vi "Load Settings from XML.vi"() -> (0 "error out":errorcluster, 3 "Settings out":T1)   [LabVIEW 2025, in "Settings Editor.lvlib"]
doc: "Attempts to load previous user specified settings from an XML file.\n\nThis VI will not generate an error. If a suitable XML file can't be loaded and parsed then it will simply return the default settings.\n_____\nBased on DQMH Dev Tools: Project Template 7.1.0.1503."
uses:
  Settings Editor.lvlib
  Settings--cluster.ctl
  <vilib>/Utility/xml.llb/Read From XML File(string).vi
  Test Meta Data.ctl
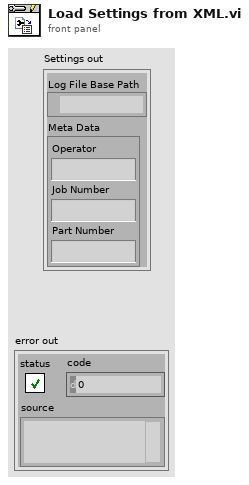
[diagram p1: front panel]
types:
  T1 = typedef "Settings Editor.lvlib/Settings--cluster.ctl" = cluster{"Log File Base Path":path, "Meta Data":T2}
  T2 = typedef "Test Meta Data.ctl" = cluster{"Operator":string, "Job Number":string, "Part Number":string}
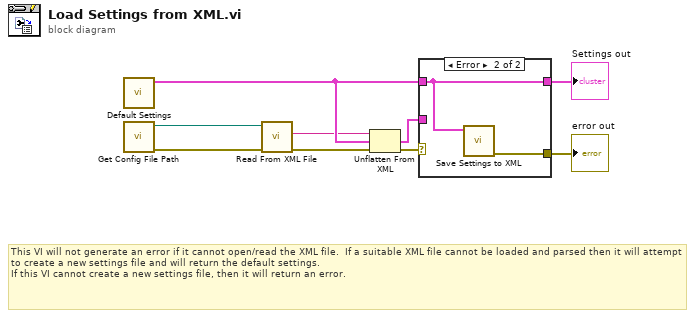
[diagram p0: block diagram]
diagram:
  # "This VI will not generate an error if it cannot open/read the XML file.  If a suitable XML file cannot be loaded and parsed then it will attempt to create a new settings file and will return the default settings.\nIf this VI cannot create a new settings file, then it will return an error."
  n1 = call "Default Settings.vi"() -> ("Default Settings"=w7:T1)  [unwired: 11 in]
  n2 = call "Get Config File Path.vi"() -> ("error out"=w3:errorcluster, "XML File Path"=w4:path)  [unwired: 10 in]
  n3 = call-poly <vilib>:"Read From XML File.vi"("error in (no error)"=w3, "XML File Path"=w4) -> ("error out"=w5:errorcluster, "XML Elements"=w6:string)  [unwired: 7 in, 1 out]
  n4 = Unflatten From XML(xml string=w6, type=w7, error in (no error)=w5) -> (value=w1:T1, error out=w2:errorcluster)
  n5 = case shown="Error" w2 {
    tunnel: [w10 w12] -> w8
    tunnel: w7 -> [_ w12]
    tunnel: w1 -> [w10 _]
    tunnel: [_ w11] -> w9
    frame No Error {
    }
    frame Error {
      n6 = call "Save Settings to XML.vi"("Settings"=w12) -> ("error out"=w11:errorcluster)  [unwired: 10 in]
    }
  }
  "error out" <- w9
  "Settings out" <- w8
